vi "PWMexample.vi"() -> ()   [LabVIEW 2020]
uses:
  <vilib>/Platform/TimedLoop/XDataNode/timing_clust.ctl
  <vilib>/Platform/TimedLoop/XDataNode/nitl_modes.ctl
  <vilib>/Platform/TimedLoop/XDataNode/wakeup.ctl
  <vilib>/platform/TimedLoop/XDataNode/XDataNode.xnode
  <vilib>/Platform/TimedLoop/XDataNode/XDNodeRunTimeDep.lvlib
panel:
  out "ON":bool=TRUE
  out "Waveform Chart":cluster{dbl, dbl, dbl}(graph)={250.0, 70.0, 1.0}
  in  "stop":bool
  in  "Duty Cycle [0-100%]":dbl(slide)=50.0 scale=0.0..100.0
  in  "Period [ms]":dbl=500.0
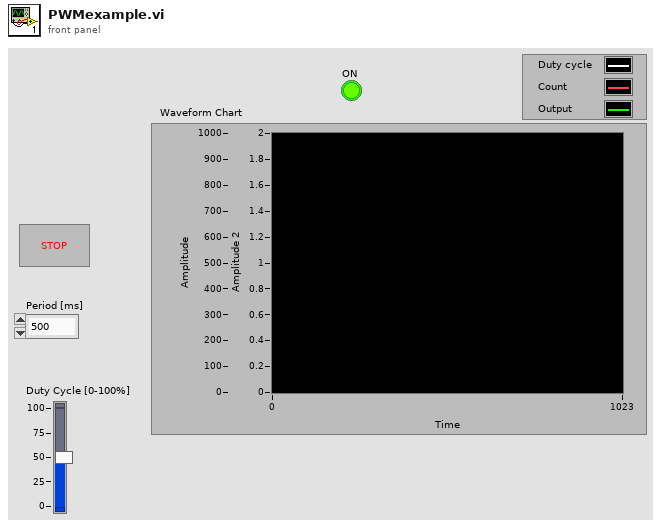
[diagram p1: front panel]
types:
  T1 = typedef "XDNodeRunTimeDep.lvlib/timing_clust.ctl" = cluster{"Expected End [f-1]":u64, "Actual End [f-1]":u64, "Finished Late? [f-1]":bool, "Expected End [i-1]":u64, "Actual End [i-1]":u64, "Finished Late? [i-1]":bool, "Expected Start [i]":u64, "Actual Start [i]":u64, "Expected Start [f]":u64, "Actual Start [f]":u64, "Source Name":string, "Structure Name":string, "Period":i64, "Deadline":i64, "Offset":i64, "Start":i64, "Priority":i32, "Timeout":i32, "Mode":T2, "Wakeup Reason":T3, "Error":errorcluster, "Source Type":string, "Secondary Source Type":string, "Global End Time":u64, "Global Start Time":u64, "Frame Duration":u64, "Iteration Duration":u64, "Assigned CPU":i32, "I/O Scan Engine Mode":u32}
  T2 = typedef "XDNodeRunTimeDep.lvlib/nitl_modes.ctl" = enum32{"No Change", "Process missed periods, maintain original phase", "Discard missed periods, maintain original phase", "Process missed periods, ignore original phase", "Discard missed periods, ignore original phase"}
  T3 = typedef "XDNodeRunTimeDep.lvlib/wakeup.ctl" = enum32{"Normal", "Aborted", "Asynchronous wakeup", "Timing source error", "Timed loop error", "Timeout"}
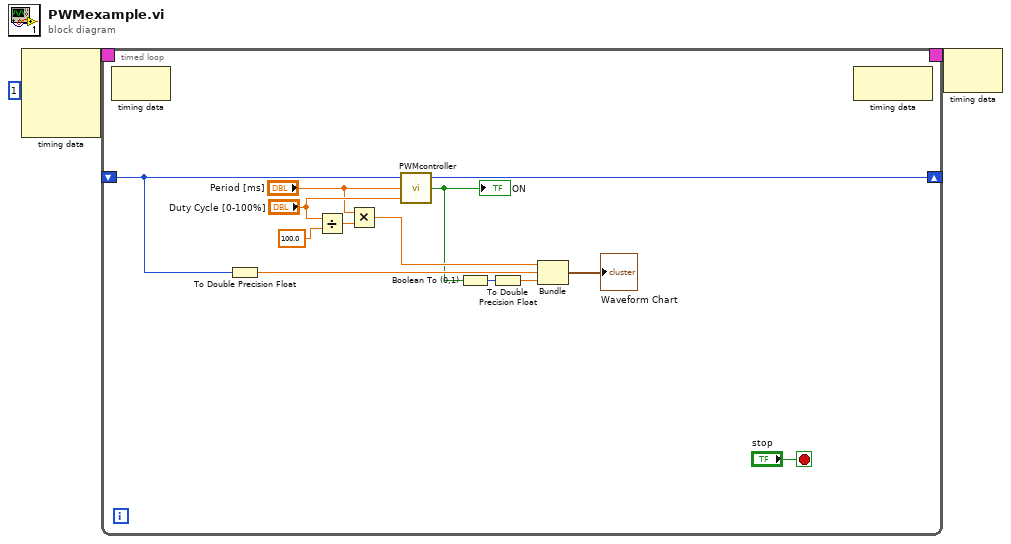
[diagram p0: block diagram]
diagram:
  n1 = node-c288(i64 1 ("Period")) -> (w3:T1)  [unwired: 3 in]
  n2 = timed-loop {
    timing: w3 -> [_]
    timing-out: [_] -> w2
    shift-right: [w16] -> _
    shift-left: _ -> [w15]
    stop <- "stop" stop-if-true
    n3 = node-c288() -> ()  [unwired: 1 in, 1 out]
    n4 = To Double Precision Float(number=w15) -> (double precision float=w14:dbl)
    n5 = Divide(x="Duty Cycle [0-100%]", y=100.0) -> (x/y=w9:dbl)
    n6 = Multiply(x="Period [ms]", y=w9) -> (x*y=w7:dbl)
    n7 = call "PWMcontroller.vi"("Duty Cycle [0-100%]"="Duty Cycle [0-100%]", "Period [ms]"="Period [ms]", "Count in"=w15) -> ("State"=w6:bool, "Count out"=w16:u32)  [unwired: 1 in]
    "ON" <- w6
    n8 = Boolean To (0,1)(Boolean=w6) -> (0, 1=w5:i16)
    n9 = To Double Precision Float(number=w5) -> (double precision float=w4:dbl)
    n10 = Bundle(w7, w14, w4) -> (→"Waveform Chart":cluster{dbl, dbl, dbl})  [unwired: 1 in]
    n11 = node-c288() -> ()  [unwired: 1 in, 1 out]
  }
  n12 = node-c288(w2) -> ()  [unwired: 1 out]
